vi "Execute.vi"(8 "error in (no error)":errorcluster, 11 "reference in":refnum<class "GarageDoorOpenCommand.lvclass">) -> (0 "error out":errorcluster, 3 "reference in":refnum<class "GarageDoorOpenCommand.lvclass">)   [LabVIEW 2020, in "GarageDoorOpenCommand.lvclass"]
uses:
  GarageDoorOpenCommand.lvclass
  GarageDoor_class/GarageDoor.lvclass
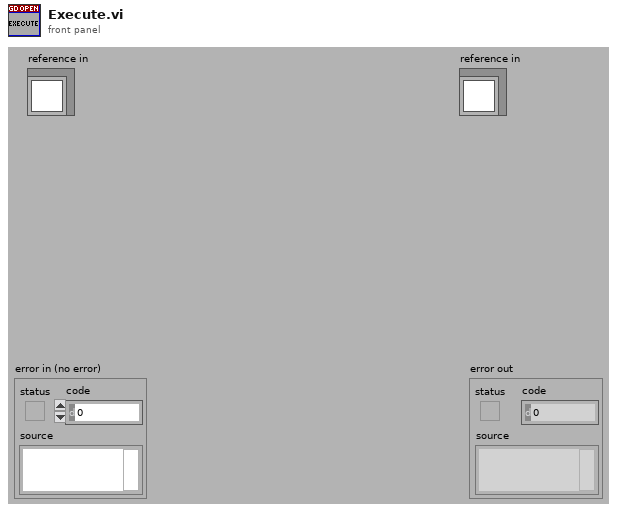
[diagram p1: front panel]
types:
  T1 = typedef "GarageDoorOpenCommand.lvclass/ObjectAttributes.ctl" = cluster{"GarageDoor":refnum<class "GarageDoor.lvclass">}
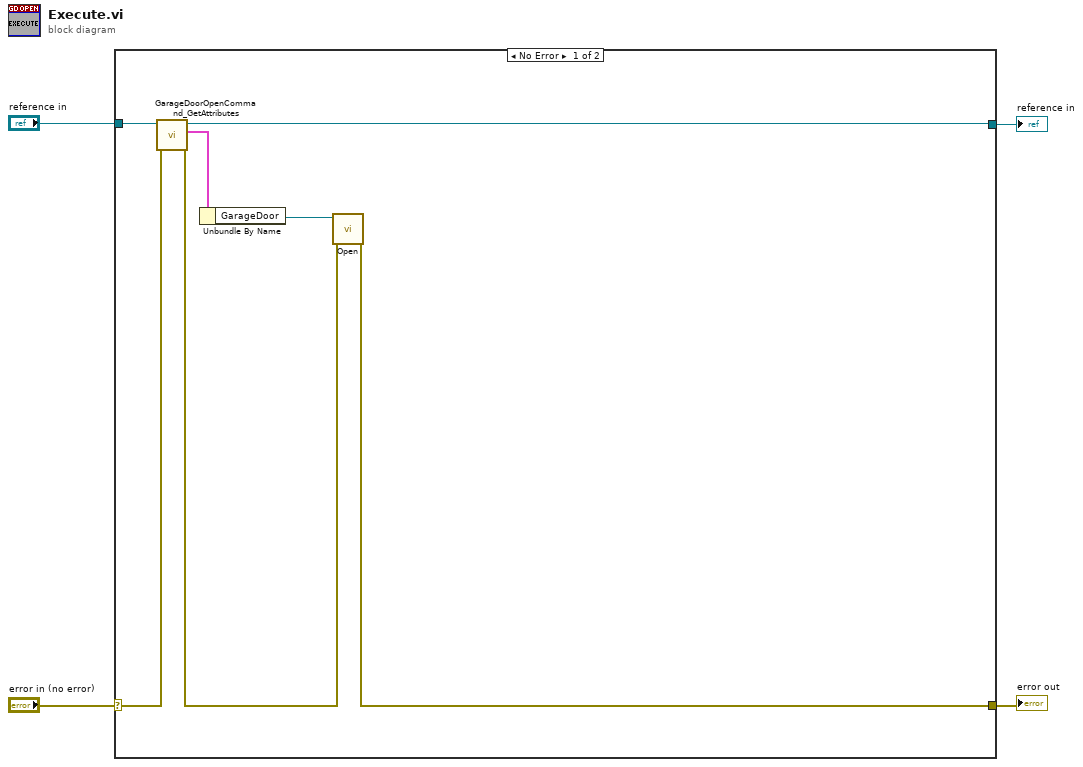
[diagram p0: block diagram]
diagram:
  n1 = case shown="No Error" "error in (no error)" {
    selector: "error in (no error)" -> [w10 w13]
    tunnel: [w5 w13] -> w3
    tunnel: [w8 w12] -> w1
    tunnel: "reference in" -> [w11 w12]
    frame No Error {
      n2 = call "GarageDoorOpenCommand_GetAttributes.vi"("error in (no error)"=w10, "reference in"=w11) -> ("error out"=w6:errorcluster, "Data"=w9:T1, "reference out"=w8:refnum<class "GarageDoorOpenCommand.lvclass">)  [unwired: 6 in, 1 out]
      n3 = Unbundle By Name(w9) -> ("GarageDoor"=w7:refnum<class "GarageDoor.lvclass">)
      n4 = call-dynamic "Open.vi"("error in (no error)"=w6, "reference in"=w7) -> ("error out"=w5:errorcluster)  [unwired: 8 in, 1 out]
    }
    frame Error {
    }
  }
  "error out" <- w3
  "reference in" <- w1
